vi "niRFSysCalReader Create Interpolation Table.vi"(8 "error in":errorcluster, 11 "niRFSysCalReader Handle":T1) -> (0 "error out":errorcluster, 2 "Interpolation Table":dbl[][][](array[numeric]), 3 "niRFSysCalReader Handle out":T1)   [LabVIEW 2018, in "niRFSysCalReader.lvlib"]
uses:
  niRFSysCalReader.lvlib
  INCLUDES/niRFSysCalReader Handle.ctl
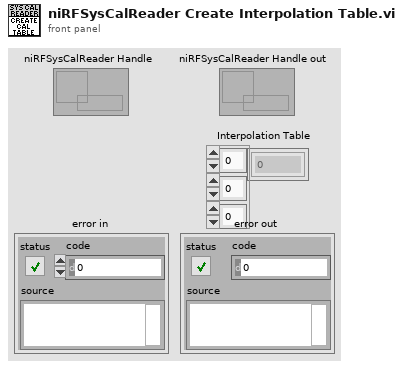
[diagram p1: front panel]
types:
  T1 = typedef "niRFSysCalReader.lvlib/niRFSysCalReader Handle.ctl" = refnum<data-value>
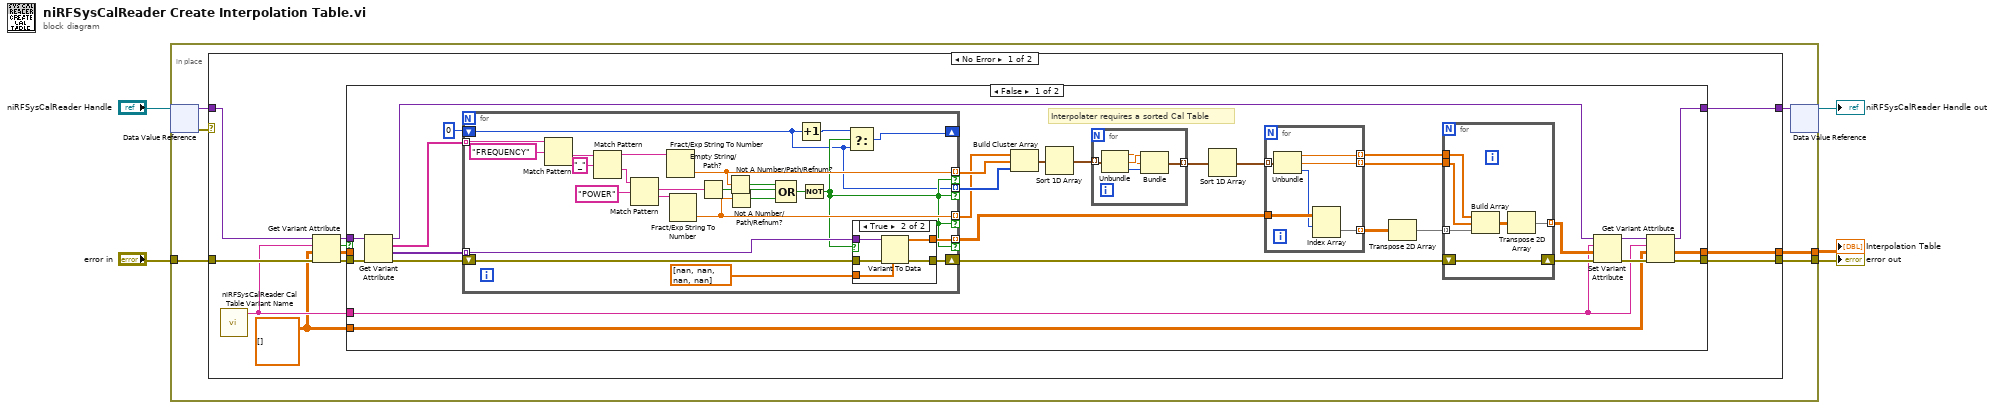
[diagram p0: block diagram]
diagram:
  n1 = in-place {
    in-place-border: [w11] -> w5
    in-place-border: "error in" -> [w7]
    in-place-border: [w9] -> w3
    n2 = in-place-dvr #1("niRFSysCalReader Handle") -> (w8:variant, w6:errorcluster)
    n3 = case shown="No Error" w6 {
      tunnel: [w22 _] -> w11
      tunnel: [w21 w103] -> w10
      tunnel: [w20 w102] -> w9
      tunnel: w8 -> [w19 w103]
      tunnel: w7 -> [w14 w102]
      frame No Error {
        w12 = dbl[][][] []
        n4 = call "niRFSysCalReader Cal Table Variant Name.vi"() -> ("Calibration Table Name"=w13:string)  [unwired: 11 in]
        n5 = Get Variant Attribute(Variant=w19, name=w13, default value (empty Variant)=w12, error in=w14) -> (duplicate Variant=w17:variant, found=w16:bool, value=w15:dbl[][][], error out=w18:errorcluster)
        n6 = case shown="False" w16 {
          tunnel: [w24 w99] -> w22
          tunnel: [w26 w100] -> w21
          tunnel: [w28 w101] -> w20
          tunnel: w18 -> [w48 w101]
          tunnel: w17 -> [w47 w100]
          tunnel: w15 -> [_ w99]
          tunnel: w13 -> [w25 _]
          tunnel: w12 -> [w23 _]
          frame False {
            # "Interpolater requires a sorted Cal Table"
            n7 = Get Variant Attribute(Variant=w47, error in=w48) -> (duplicate Variant=w29:variant, names=w51:string[], values=w50:variant[], error out=w49:errorcluster)  [unwired: 2 in]
            n8 = for {
              tunnel: [w92] -> w44 mode=indexing if=w72
              tunnel: [w78] -> w43 mode=indexing if=w72
              shift-right: [w90] -> w35
              shift-left: w49 -> [w91]
              tunnel: [w89] -> w38 mode=indexing if=w72
              tunnel: w50 -> [w88] mode=indexing
              tunnel: w51 -> [w81] mode=indexing
              tunnel: [w69] -> w46 mode=indexing if=w72
              shift-right: [w70] -> _
              shift-left: 0 -> [w69]
              n9 = Match Pattern(string=w81, regular expression="FREQUENCY") -> (after substring=w83:string)  [unwired: 1 in, 3 out]
              n10 = Match Pattern(string=w83, regular expression="_" ("string")) -> (before substring=w80:string, after substring=w85:string)  [unwired: 1 in, 2 out]
              n11 = Match Pattern(string=w85, regular expression="POWER" ("string")) -> (match substring=w77:string, after substring=w79:string)  [unwired: 1 in, 2 out]
              n12 = Fract/Exp String To Number(string=w80) -> (number=w92:dbl)  [unwired: 3 in, 1 out]
              n13 = Fract/Exp String To Number(string=w79) -> (number=w78:dbl)  [unwired: 3 in, 1 out]
              n14 = Empty String/Path?(string/path=w77) -> (empty?=w75:bool)
              n15 = Not A Number/Path/Refnum?(number/path/refnum=w92) -> (NaN/Path/Refnum?=w76:bool)
              n16 = Not A Number/Path/Refnum?(number/path/refnum=w78) -> (NaN/Path/Refnum?=w74:bool)
              n17 = Compound Arithmetic op=OR(w76, w75, w74) -> (w73:bool)
              n18 = Increment(x=w69) -> (x+1=w71:i32)
              n19 = Not(x=w73) -> (.not. x?=w72:bool)
              n20 = Select(t=w71, s=w72, f=w69) -> (s? t:f=w70:i32)
              n21 = case shown="True" w72 {
                tunnel: w91 -> [w93 w98]
                tunnel: [w93 w97] -> w90
                tunnel: [_ w96] -> w89
                tunnel: w88 -> [_ w95]
                tunnel: dbl[] [nan, nan, nan, nan] -> [_ w94]
                frame False {
                }
                frame True {
                  n22 = Variant To Data(error in=w98, type=w94, Variant=w95) -> (data=w96:dbl[], error out=w97:errorcluster)
                }
              }
            }
            n23 = Build Cluster Array(w43, w44, w46) -> (w45:cluster{dbl, dbl, i32}[])
            n24 = Sort 1D Array(array=w45) -> (sorted array=w42:cluster{dbl, dbl, i32}[])
            n25 = for {
              tunnel: w42 -> [w68] mode=indexing
              tunnel: [w64] -> w41 mode=indexing
              n26 = Unbundle(w68) -> (w66:dbl, w67:dbl, w65:i32)
              n27 = Bundle(w67, w66, w65) -> (w64:cluster{dbl, dbl, i32})  [unwired: 1 in]
            }
            n28 = Sort 1D Array(array=w41) -> (sorted array=w40:cluster{dbl, dbl, i32}[])
            n29 = for {
              tunnel: w40 -> [w63] mode=indexing
              tunnel: w38 -> [w62]
              tunnel: [w61] -> w34 mode=indexing
              tunnel: [w60] -> w37 mode=indexing
              tunnel: [w59] -> w36 mode=indexing
              n30 = Unbundle(w63) -> (w60:dbl, w59:dbl, w58:i32)
              n31 = Index Array(array=w62, index (row)=w58) -> (element=w61:dbl[])  [unwired: 1 in]
            }
            n32 = Transpose 2D Array(2D array=w34) -> (transposed array=w33:dbl[][])
            n33 = for {
              tunnel: w37 -> [w55]
              tunnel: w36 -> [w54]
              shift-right: [w53] -> w32
              shift-left: w35 -> [w53]
              tunnel: w33 -> [w57] mode=indexing
              tunnel: [w52] -> w30 mode=indexing
              n34 = Build Array(w55, w54, w57) -> (w56:dbl[][])
              n35 = Transpose 2D Array(2D array=w56) -> (transposed array=w52:dbl[][])
            }
            n36 = Set Variant Attribute(Variant=w29, name=w25, value=w30, error in=w32) -> (Variant out=w27:variant, error out=w31:errorcluster)  [unwired: 1 out]
            n37 = Get Variant Attribute(Variant=w27, name=w25, default value (empty Variant)=w23, error in=w31) -> (duplicate Variant=w26:variant, value=w24:dbl[][][], error out=w28:errorcluster)  [unwired: 1 out]
          }
          frame True {
          }
        }
      }
      frame Error {
      }
    }
    n38 = in-place-dvr #1(w10) -> (→"niRFSysCalReader Handle out":T1)  [unwired: 1 out]
  }
  "Interpolation Table" <- w5
  "error out" <- w3
